vi "Set Parameter.vi"(6 "Value":string, 8 "error in (no error)":errorcluster, 9 "Type":T1, 10 "Name":string, 11 "IED in":refnum<class "IED.lvclass">) -> (0 "error out":errorcluster, 3 "IED out":refnum<class "IED.lvclass">)   [LabVIEW 2015, in "IED Actor.lvlib" / "IED.lvclass"]
uses:
  IED.lvclass
  SCADA Core/SCADA/Controls/Parameter Type.ctl
  <vilib>/ActorFramework/Actor/Actor.lvclass/Actor.ctl
  IED.lvclass/IED.ctl
  SCADA Core/SCADA Abstract Messages/Set Device Parameter Status Msg/Set Device Parameter Status.ctl
  <vilib>/Utility/error.llb/DialogType.ctl
  SCADA Core/SCADA Response Messages/Return Parameter Status Msg/Return Parameter Status Msg.lvclass/Return Parameter Status Msg.ctl
  <vilib>/ActorFramework/Message Enqueuer/Message Enqueuer.lvclass/Message Enqueuer.ctl
  <vilib>/NI/Tools/Keyed Array/Map String.vi
  <vilib>/ActorFramework/Message Enqueuer/Enqueue.vi
  <vilib>/NI/Tools/String/Get Case Matching.vi
  <vilib>/ActorFramework/Message Priority Queue/Priority Enqueue.vi
  SCADA Core/SCADA Response Messages/Return Parameter Status Msg/Return Parameter Status Msg.lvclass
  <vilib>/Modbus/master/Modbus Master.lvclass
  <vilib>/NI/Tools/Keyed Array/Tools_KeyedArray.lvlib
  Utilities/Message Strings.llb/Message String Utilities.lvlib
  <vilib>/ActorFramework/Actor/Actor.lvclass
  SCADA Core/SCADA Abstract Messages/Set Device Parameter Status Msg/Set Device Parameter Status Msg.lvclass
  SCADA Core/SCADA/SCADA.lvclass
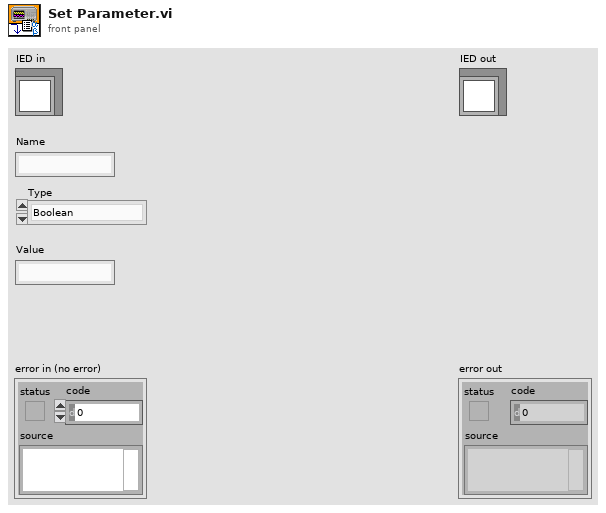
[diagram p1: front panel]
types:
  T1 = typedef "SCADA Core.lvlib/SCADA.lvclass/Parameter Type.ctl" = enum8{"Boolean", "U16", "U32", "I32", "Double", "String"}
  T2 = typedef "SCADA Core.lvlib/Set Device Parameter Status Msg.lvclass/Set Device Parameter Status.ctl" = enum16{"Success", "Failure"}
  T3 = typedef "Tools_KeyedArray.lvlib/KeyedArray.ctl" = cluster{"keys":string[], "values":string[]}
  T4 = typedef "DialogType.ctl" = u16
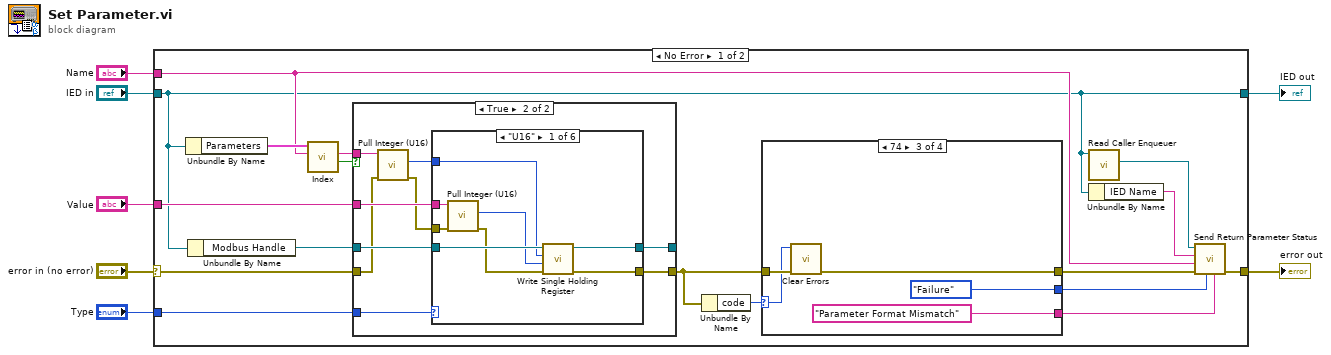
[diagram p0: block diagram]
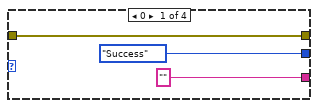
[diagram p2: hidden frame]
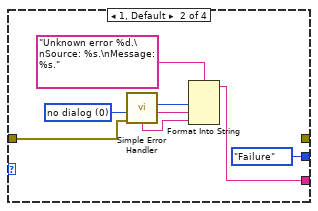
[diagram p3: hidden frame]
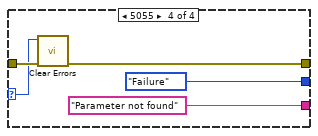
[diagram p4: hidden frame]
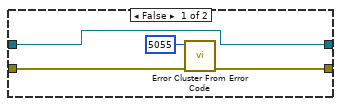
[diagram p5: hidden frame]
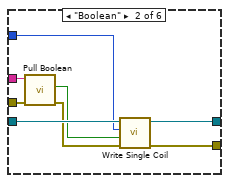
[diagram p6: hidden frame]
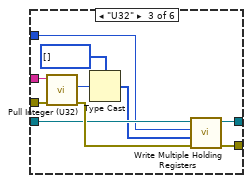
[diagram p7: hidden frame]
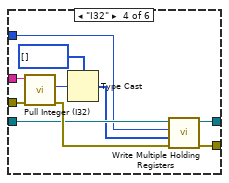
[diagram p8: hidden frame]
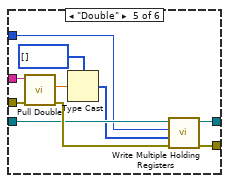
[diagram p9: hidden frame]
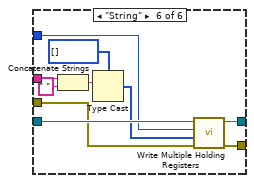
[diagram p10: hidden frame]
diagram:
  n1 = case shown="No Error" "error in (no error)" {
    selector: "error in (no error)" -> [w10 w116]
    tunnel: [w17 w116] -> w6
    tunnel: [w11 w115] -> w4
    tunnel: "IED in" -> [w11 w115]
    tunnel: "Name" -> [w14 _]
    tunnel: "Type" -> [w21 _]
    tunnel: "Value" -> [w20 _]
    frame No Error {
      n2 = Unbundle By Name(w11) -> ("Parameters"=w24:T3)
      n3 = Unbundle By Name(w11) -> ("Modbus Handle"=w9:refnum<class "Modbus Master.lvclass">)
      n4 = call <vilib>:"Index.vi"("key"=w14, "array in"=w24) -> ("valid key"=w23:bool, "value"=w22:string)  [unwired: 3 in, 1 out]
      n5 = case shown="True" w23 {
        tunnel: w22 -> [_ w58]
        tunnel: w21 -> [_ w57]
        tunnel: w20 -> [_ w56]
        tunnel: w9 -> [w46 w55]
        tunnel: w10 -> [w48 w54]
        tunnel: [w49 w51] -> w8
        tunnel: [w46 w50] -> _
        frame False {
          n6 = call <vilib>:"Error Cluster From Error Code.vi"("error in (no error)"=w48, "error code (0)"=5055) -> ("error out"=w49:errorcluster)  [unwired: 7 in]
        }
        frame True {
          n7 = call "Pull Integer (U16).vi"("error in (no error)"=w54, "String in"=w58) -> ("error out"=w53:errorcluster, "Integer out"=w52:u16)  [unwired: 7 in, 1 out]
          n8 = case shown="\"U16\"" w57 {
            tunnel: w56 -> [w66 w74 w84 w94 w104 w108]
            tunnel: w55 -> [w65 w73 w80 w90 w100 w113]
            tunnel: w53 -> [w64 w72 w83 w93 w103 w109]
            tunnel: w52 -> [w62 w70 w79 w89 w99 w112]
            tunnel: [w61 w69 w81 w91 w101 w114] -> w51
            tunnel: [w59 w67 w75 w85 w95 w105] -> w50
            frame "U16" {
              n9 = call "Pull Integer (U16).vi"("error in (no error)"=w64, "String in"=w66) -> ("error out"=w63:errorcluster, "Integer out"=w60:u16)  [unwired: 7 in, 1 out]
              n10 = call-dynamic "Write Single Holding Register.vi"("error in (no error)"=w63, "holding register value"=w60, "address"=w62, "Modbus master in"=w65) -> ("error out"=w61:errorcluster, "Modbus master out"=w59:refnum<class "Modbus Master.lvclass">)  [unwired: 6 in]
            }
            frame "Boolean" {
              n11 = call "Pull Boolean.vi"("error in (no error)"=w72, "String in"=w74) -> ("error out"=w71:errorcluster, "Boolean out"=w68:bool)  [unwired: 7 in, 1 out]
              n12 = call-dynamic "Write Single Coil.vi"("error in (no error)"=w71, "coil value"=w68, "address"=w70, "Modbus master in"=w73) -> ("error out"=w69:errorcluster, "Modbus master out"=w67:refnum<class "Modbus Master.lvclass">)  [unwired: 6 in]
            }
            frame "U32" {
              n13 = call "Pull Integer (U32).vi"("error in (no error)"=w83, "String in"=w84) -> ("error out"=w82:errorcluster, "Integer out"=w78:u32)  [unwired: 7 in, 1 out]
              n14 = Type Cast(type=u16[] [] ("holding register values"), x=w78) -> (*(type *) &x=w76:u16[])
              n15 = call-dynamic "Write Multiple Holding Registers.vi"("error in (no error)"=w82, "holding register values"=w76, "starting address"=w79, "Modbus master in"=w80) -> ("error out"=w81:errorcluster, "Modbus master out"=w75:refnum<class "Modbus Master.lvclass">)  [unwired: 6 in]
            }
            frame "I32" {
              n16 = call "Pull Integer (I32).vi"("error in (no error)"=w93, "String in"=w94) -> ("error out"=w92:errorcluster, "Integer out"=w88:i32)  [unwired: 7 in, 1 out]
              n17 = Type Cast(type=u16[] [] ("holding register values"), x=w88) -> (*(type *) &x=w86:u16[])
              n18 = call-dynamic "Write Multiple Holding Registers.vi"("error in (no error)"=w92, "holding register values"=w86, "starting address"=w89, "Modbus master in"=w90) -> ("error out"=w91:errorcluster, "Modbus master out"=w85:refnum<class "Modbus Master.lvclass">)  [unwired: 6 in]
            }
            frame "Double" {
              n19 = call "Pull Double.vi"("error in (no error)"=w103, "String in"=w104) -> ("error out"=w102:errorcluster, "Double out"=w98:dbl)  [unwired: 7 in, 1 out]
              n20 = Type Cast(type=u16[] [] ("holding register values"), x=w98) -> (*(type *) &x=w96:u16[])
              n21 = call-dynamic "Write Multiple Holding Registers.vi"("error in (no error)"=w102, "holding register values"=w96, "starting address"=w99, "Modbus master in"=w100) -> ("error out"=w101:errorcluster, "Modbus master out"=w95:refnum<class "Modbus Master.lvclass">)  [unwired: 6 in]
            }
            frame "String" {
              n22 = Concatenate Strings(w108, " " ("string")) -> (w107:string)
              n23 = Type Cast(type=u16[] [] ("holding register values"), x=w107) -> (*(type *) &x=w110:u16[])
              n24 = call-dynamic "Write Multiple Holding Registers.vi"("error in (no error)"=w109, "holding register values"=w110, "starting address"=w112, "Modbus master in"=w113) -> ("error out"=w114:errorcluster, "Modbus master out"=w105:refnum<class "Modbus Master.lvclass">)  [unwired: 6 in]
            }
          }
        }
      }
      n25 = Unbundle By Name(w8) -> ("code"=w19:i32)
      n26 = case shown="74" w19 {
        selector: w19 -> [_ _ w39 w44]
        tunnel: w8 -> [w27 w30 w40 w45]
        tunnel: [w27 _ w38 w43] -> w18
        tunnel: [Set_Device_Parameter_Status."Success" ("Status") Set_Device_Parameter_Status."Failure" ("Status") Set_Device_Parameter_Status."Failure" ("Status") Set_Device_Parameter_Status."Failure" ("Status")] -> w13
        tunnel: ["" w29 "Parameter Format Mismatch" "Parameter not found"] -> w12
        frame 0 {
        }
        frame 1, Default {
          w35 = T4 0 items=["no dialog", "OK message", "continue or stop message", "OK message + warnings", "continue/stop + warnings"] ("type of dialog (OK msg:1)")
          n27 = call <vilib>:"Simple Error Handler.vi"("type of dialog (OK msg:1)"=w35, "error in (no error)"=w30) -> ("code out"=w33:i32, "source out"=w32:string, "message"=w31:string)  [unwired: 3 in, 2 out]
          n28 = Format Into String(format string="Unknown error %d.\nSource: %s.\nMessage: %s." ("Error String"), w33, w32, w31) -> (resulting string=w29:string)  [unwired: 2 in, 1 out]
        }
        frame 74 {
          n29 = call <vilib>:"Clear Errors.vi"("error in (no error)"=w40, "specific error code to clear (0: all)"=w39) -> ("error out"=w38:errorcluster)  [unwired: 4 in, 1 out]
        }
        frame 5055 {
          n30 = call <vilib>:"Clear Errors.vi"("error in (no error)"=w45, "specific error code to clear (0: all)"=w44) -> ("error out"=w43:errorcluster)  [unwired: 4 in, 1 out]
        }
      }
      n31 = call <vilib>:"Read Caller Enqueuer.vi"("Actor"=w11) -> ("Caller Enqueuer"=w16:refnum<class "Message Enqueuer.lvclass">)  [unwired: 10 in]
      n32 = Unbundle By Name(w11) -> ("IED Name"=w15:string)
      n33 = call "Send Return Parameter Status.vi"("error"=w12, "Status"=w13, "error in (no error)"=w18, "Parameter Name"=w14, "IED Name"=w15, "Message Enqueuer"=w16) -> ("error out"=w17:errorcluster)  [unwired: 4 in, 1 out]
    }
    frame Error {
    }
  }
  "error out" <- w6
  "IED out" <- w4
